vi "_unloadStage.vi"(8 "error in (no error)":errorcluster, 11 "_delayStageBase in":refnum<class "_delayStageBase.lvclass">) -> (0 "error out":errorcluster, 3 "_delayStageBase out":refnum<class "_delayStageBase.lvclass">)   [LabVIEW 2019, in "_delayStageBase.lvclass"]
uses:
  _delayStageBase.lvclass
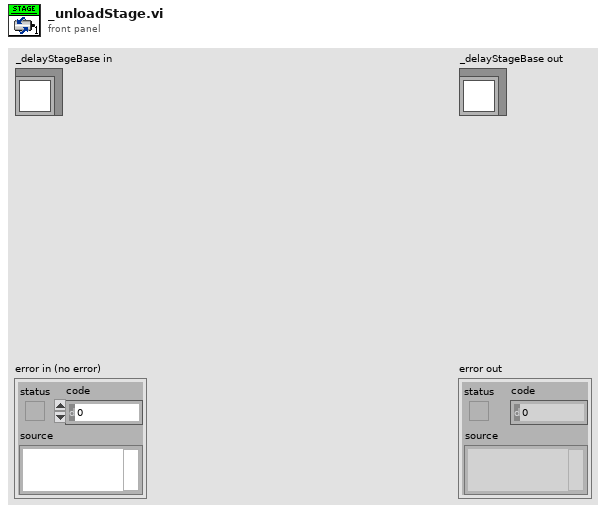
[diagram p1: front panel]
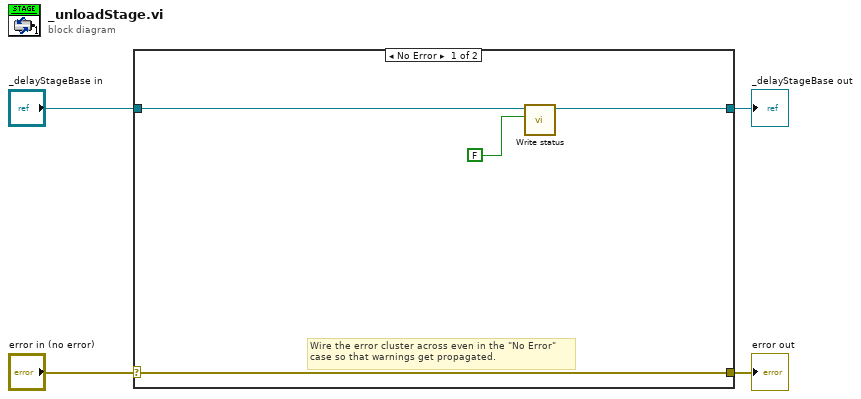
[diagram p0: block diagram]
diagram:
  n1 = case shown="No Error" "error in (no error)" {
    selector: "error in (no error)" -> [w8 w10]
    tunnel: [w8 w10] -> w3
    tunnel: [w6 w9] -> w1
    tunnel: "_delayStageBase in" -> [w7 w9]
    frame No Error {
      # "Wire the error cluster across even in the \"No Error\"\ncase so that warnings get propagated."
      n2 = call-dynamic "Write status.vi"("status"=FALSE, "_delayStageBase in"=w7) -> ("_delayStageBase out"=w6:refnum<class "_delayStageBase.lvclass">)  [unwired: 8 in, 1 out]
    }
    frame Error {
    }
  }
  "error out" <- w3
  "_delayStageBase out" <- w1
